vi "sendMessage.vi"(8 "error in (no error)":errorcluster, 10 "message":string, 11 "AlCS in":refnum<class "AlCS.lvclass">) -> (0 "error out":errorcluster, 3 "AlCS out":refnum<class "AlCS.lvclass">)   [LabVIEW 2016, in "AlCS.lvclass"]
uses:
  AlCS.lvclass
  AlCS.lvclass/AlCS.ctl
  ts_labview_tcp/TCPClient/TCPClient.lvclass
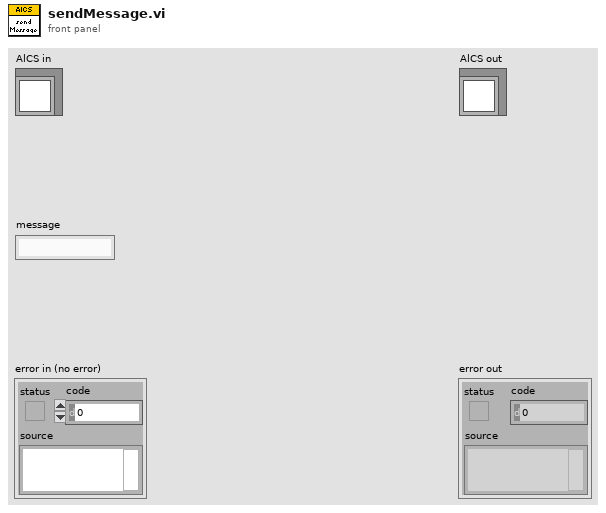
[diagram p1: front panel]
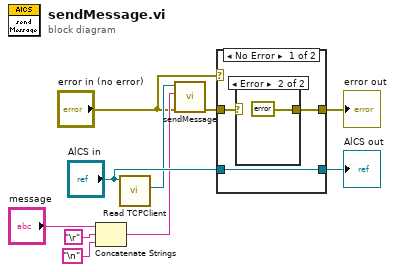
[diagram p0: block diagram]
diagram:
  n1 = Concatenate Strings("message", "\r", "\n") -> (w3:string)
  n2 = call "Read TCPClient.vi"("AlCS in"="AlCS in") -> ("TCPClient.lvclass"=w4:refnum<class "TCPClient.lvclass">)  [unwired: 8 in, 2 out]
  n3 = call-dynamic "sendMessage.vi"("error in (no error)"="error in (no error)", "String"=w3, "TCPClient in"=w4) -> ("error out"=w1:errorcluster)  [unwired: 7 in, 1 out]
  n4 = case shown="No Error" "error in (no error)" {
    selector: "error in (no error)" -> [_ w16]
    tunnel: [w12 w16] -> w10
    tunnel: [w13 w17] -> w9
    tunnel: "AlCS in" -> [w13 w17]
    tunnel: w1 -> [w11 _]
    frame No Error {
      n5 = case shown="Error" w11 {
        selector: w11 -> [w14 _]
        tunnel: [w14 errorcluster {"status"=TRUE, "code"=8204, "source"="Monochromator Controller not responding"} ("error IO")] -> w12
        frame No Error {
        }
        frame Error {
        }
      }
    }
    frame Error {
    }
  }
  "error out" <- w10
  "AlCS out" <- w9
